vi "PH_Beckhoff_Application.declare digital Timing InputTags.vi"() -> (0 "Digital Inputs":T2, 1 "Description":string)   [LabVIEW 2014, in "PH_Beckhoff_Application.lvlib"]
uses:
  PH_Beckhoff_Application.lvlib
  PH_Beckhoff/PH_Beckhoff.Digital Inputs.ctl
  PH_Beckhoff/PH_Beckhoff.lvlib
panel:
  in  "Digital Input Value":T1
  out "Right Size?":bool
  # "Let this VI run to check the size!"
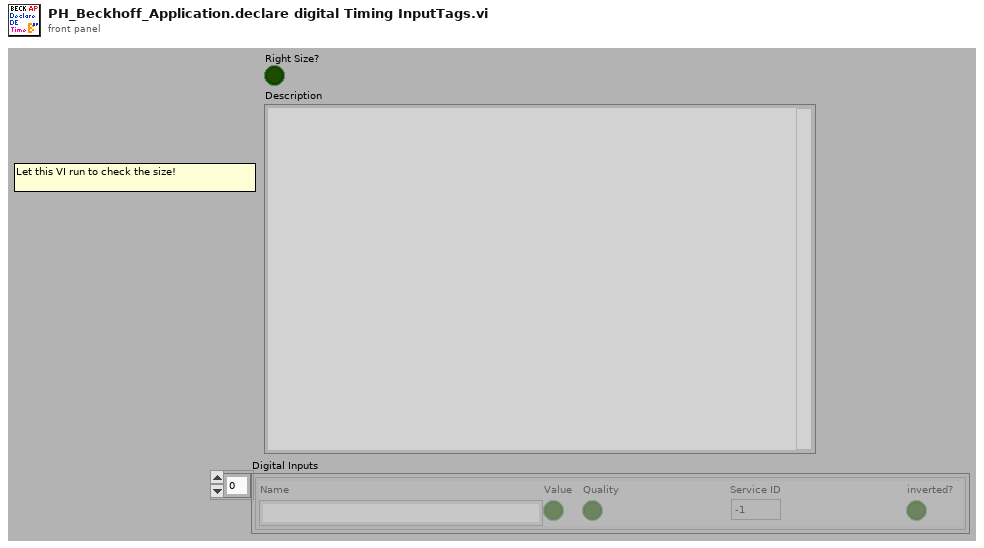
[diagram p1: front panel]
types:
  T1 = cluster{"Name":string, "Value":bool, "Quality":bool, "Service ID":i32, "inverted?":bool}
  T2 = typedef "PH_Beckhoff.lvlib/PH_Beckhoff.Digital Inputs.ctl" = cluster{"Name":string, "Value":bool, "Quality":bool, "Service ID":i32, "inverted?":bool}[]
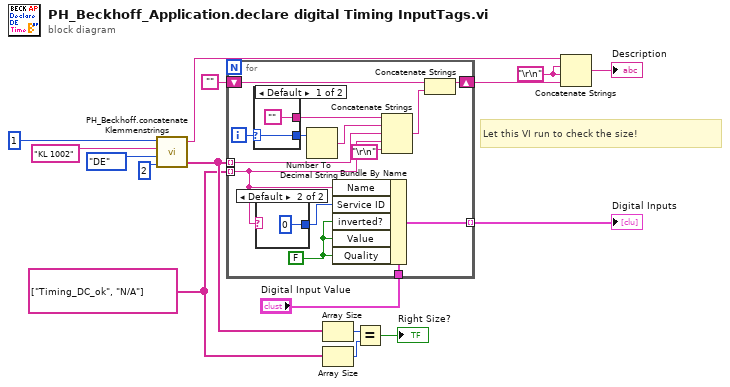
[diagram p0: block diagram]
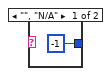
[diagram p2: hidden frame]
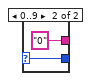
[diagram p3: hidden frame]
diagram:
  w1 = string[] ["Timing_DC_ok", "N/A"]
  w12 = "\r\n"
  # "Let this VI run to check the size!"
  n1 = call "PH_Beckhoff.concatenate Klemmenstrings.vi"("# of In- or Outputs"=2, "Type"=enum16{"AE", "AA", "DE", "DA"}."DE", "Klemmenname"="KL 1002", "Quantity"=1 ("size(s)")) -> ("concatenated string array"=w7:string[], "\"<Type>: <Quantity> x <Klemmenname>\""=w9:string)  [unwired: 1 out]
  n2 = for {
    tunnel: w1 -> [w21] mode=indexing
    tunnel: w7 -> [w26] mode=indexing
    shift-right: [w24] -> w13
    shift-left: "" -> [w23]
    tunnel: "Digital Input Value" -> [w22]
    tunnel: [w19] -> w2 mode=indexing
    i -> [w30]
    w18 = FALSE ("Quality")
    n3 = case shown="Default" w30 {
      selector: w30 -> [w33 w36]
      tunnel: [w33 w36] -> w29
      tunnel: ["" "0"] -> w28
      frame Default {
      }
      frame 0..9 {
      }
    }
    n4 = case shown="Default" w21 {
      tunnel: [-1 0] -> w20
      frame "", "N/A" {
      }
      frame Default {
      }
    }
    n5 = Number To Decimal String(number=w29) -> (decimal integer string=w27:string)  [unwired: 1 in]
    n6 = Bundle By Name(cluster=w22, "Name"=w21, "Service ID"=w20, "inverted?"=w18, "Value"=w18, "Quality"=w18) -> (w19:T1)
    n7 = Concatenate Strings(w28, w27, w26, w21, "\r\n") -> (w25:string)
    n8 = Concatenate Strings(w23, w25) -> (w24:string)
  }
  "Digital Inputs" <- w2
  n9 = Array Size(array=w7) -> (size(s)=w6:i32)
  n10 = Array Size(array=w1) -> (size(s)=w4:i32)
  n11 = Equal?(x=w6, y=w4) -> (x = y?=→"Right Size?":bool)
  n12 = Concatenate Strings(w9, w12, w12, w13) -> (→"Description":string)
